vi "LinkedIn OAuth Test.vi"() -> ()   [LabVIEW 2017]
uses:
  Oauth2/Oauth2.lvclass/Oauth2.ctl
  Oauth2.LinkedIn/Oauth2.LinkedIn.lvclass
  D:/GitHub/Oauth2/source/Oauth2/Oauth2.lvclass
  OAuthToken/Retrieve Element.vi
  Oauth2/Oauth2.lvclass
  <vilib>/LabVIEW Open Source Project/OpenURI/uri/URI.lvclass
  <vilib>/httpClient/LabVIEWHTTPClient.lvlib
  JWT/JSONWebToken.lvclass
panel:
  out "Valid JWT?":bool
  out "LinkedIn":string
  out "HTTP Response Headers":string
  in  "Client Secret":string="WPL_AP1.EOebz8MGKgZ7cZMc.BBPY/A=="
  in  "Client ID":string="781486pragll3a"
  out "LinkedIn Access Token":string
  out "error out":errorcluster
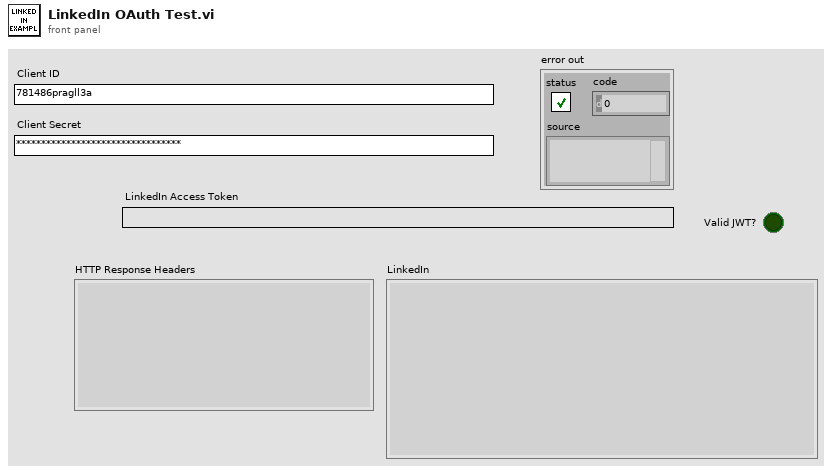
[diagram p1: front panel]
types:
  T1 = typedef "LabVIEWHTTPClient.lvlib/ClientHandle.ctl" = refnum<k1>
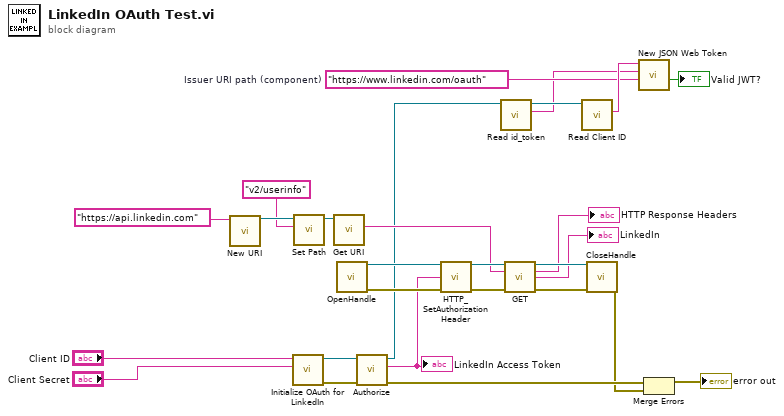
[diagram p0: block diagram]
diagram:
  w5 = "https://www.linkedin.com/oauth"  # Issuer URI path (component)
  n1 = call <vilib>:"New URI.vi"("URI"="https://api.linkedin.com" ("path")) -> ("URI"=w27:refnum<class "URI.lvclass">)  [unwired: 9 in, 1 out]
  n2 = call "Initialize OAuth for LinkedIn.vi"("Client Secret"="Client Secret", "Client ID"="Client ID") -> ("error out"=w1:errorcluster, "Oauth2.LinkedIn"=w10:refnum<class "Oauth2.LinkedIn.lvclass">)  [unwired: 8 in]
  n3 = call <vilib>:"Set Path.vi"("path"="v2/userinfo", "URI in"=w27) -> ("URI out"=w26:refnum<class "URI.lvclass">)  [unwired: 8 in, 1 out]
  n4 = call <vilib>:"Get URI.vi"("URI in"=w26) -> ("URI String"=w19:string)  [unwired: 8 in, 2 out]
  n5 = call <vilib>:"OpenHandle.vi"() -> ("client handle out"=w25:T1, "error out"=w24:errorcluster)  [unwired: 14 in]
  n6 = call "Authorize.vi"("error in (no error)"=w1, "Oauth2 in"=w10) -> ("error out"=w15:errorcluster, "Access Token"=w9:string, "Oauth2 out"=w3:refnum<class "Oauth2.lvclass">)  [unwired: 7 in]
  "LinkedIn Access Token" <- w9
  n7 = call "HTTP_SetAuthorizationHeader.vi"("Client Handle"=w25, "Access Token"=w9, "error in (no error)"=w24) -> ("client handle dup"=w23:T1, "error out"=w22:errorcluster)  [unwired: 11 in]
  n8 = call "Read id_token.vi"("Oauth2 in"=w3) -> ("id_token"=w4:string, "Oauth2 out"=w7:refnum<class "Oauth2.lvclass">)  [unwired: 8 in, 1 out]
  n9 = call <vilib>:"GET.vi"("client handle"=w23, "url"=w19, "error in (no error)"=w22) -> ("client handle out"=w21:T1, "headers"=→"HTTP Response Headers":string, "body"=→"LinkedIn":string, "error out"=w20:errorcluster)  [unwired: 9 in]
  n10 = call "Read Client ID.vi"("Oauth2 in"=w7) -> ("Client ID"=w6:string)  [unwired: 8 in, 2 out]
  n11 = call <vilib>:"CloseHandle.vi"("client handle"=w21, "error in (no error)"=w20) -> ("error out"=w13:errorcluster)  [unwired: 13 in]
  n12 = call "New JSON Web Token.vi"("Issuer URI path (component)"=w5, "Base64url JWT string"=w4, "Client ID"=w6) -> ("Valid JWT?"=→"Valid JWT?":bool)  [unwired: 3 in, 5 out]
  n13 = Merge Errors(w15, w13) -> (→"error out":errorcluster)
